vi "JSON2 speed.vi"() -> ()   [LabVIEW 2017] (continued)
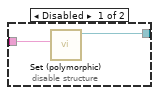
[diagram p2: hidden frame]
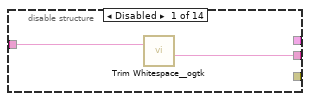
[diagram p3: hidden frame]
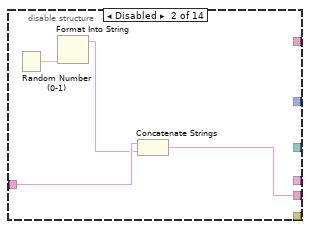
[diagram p4: hidden frame]
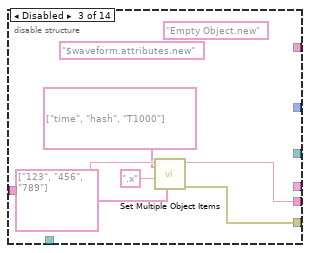
[diagram p5: hidden frame]
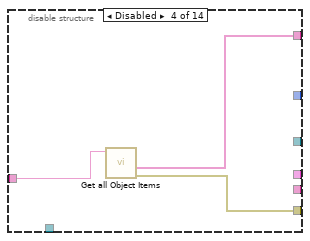
[diagram p6: hidden frame]
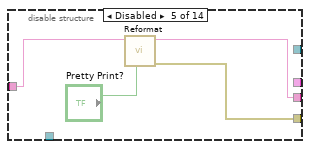
[diagram p7: hidden frame]
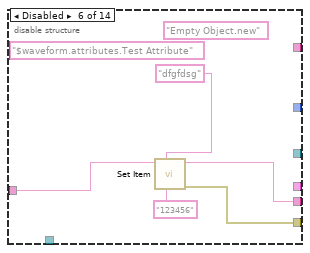
[diagram p8: hidden frame]
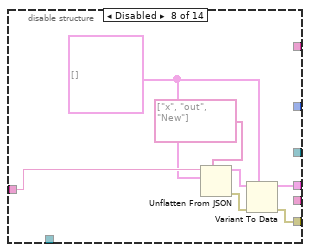
[diagram p9: hidden frame]
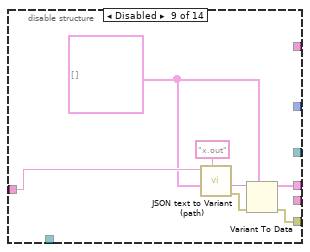
[diagram p10: hidden frame]
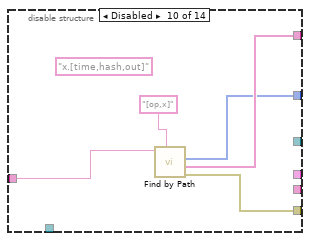
[diagram p11: hidden frame]
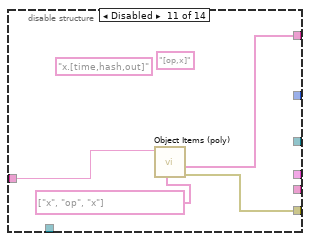
[diagram p12: hidden frame]
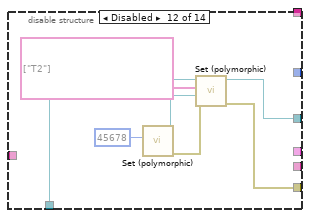
[diagram p13: hidden frame]
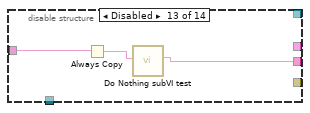
[diagram p14: hidden frame]
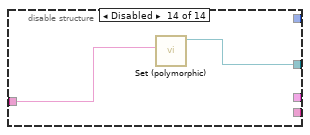
[diagram p15: hidden frame]
\\n[caliper] [performing additional measurement with scale 1.00]\\n[caliper] [running trial with 1623823839 reps]\\n[caliper] [starting measured section]\\n[caliper] [done measured section]\\n[caliper] [took 0.61 nanoseconds per rep]\\n\"}}},{\"k\":{\"variables\":{\"vm\":\"java\",\"trial\":\"0\",\"benchmark\":\"ToArray\",\"size\":\"300\"}},\"v\":{\"measurementSetMap\":{\"TIME\":{\"measurements\":[{\"raw\":239.58869988386775,\"processed\":239.58869988386775,\"unitNames\":{\"ns\":1,\"s\":1000000000,\"ms\":1000000,\"us\":1000}},{\"raw\":235.73190589527383,\"processed\":235.73190589527383,\"unitNames\":{\"ns\":1,\"s\":1000000000,\"ms\":1000000,\"us\":1000}},{\"raw\":237.79040875271875,\"processed\":237.79040875271875,\"unitNames\":{\"ns\":1,\"s\":1000000000,\"ms\":1000000,\"us\":1000}}],\"unitNames\":{\"ns\":1,\"s\":1000000000,\"ms\":1000000,\"us\":1000},\"systemOutCharCount\":0,\"systemErrCharCount\":0}},\"eventLogMap\":{\"TIME\":\"starting Scenario{vm\\u003djava, trial\\u003d0, benchmark\\u003dToArray, size\\u003d300}\\n[caliper] [starting warmup]\\n[caliper] [starting measured section]\\n[caliper] [done measured section]\\n[caliper] [starting measured section]\\n[caliper] [done measured section]\\n[caliper] [starting measured section]\\n[caliper] [done measured section]\\n[caliper] [starting measured section]\\n[caliper] [done measured section]\\n[caliper] [starting measured section]\\n[caliper] [done measured section]\\n[caliper] [starting measured section]\\n[caliper] [done measured section]\\n[caliper] [starting measured section]\\n[caliper] [done measured section]\\n[caliper] [starting measured section]\\n[caliper] [done measured section]\\n[caliper] [starting measured section]\\n[caliper] [done measured section]\\n[caliper] [starting measured section]\\n[caliper] [done measured section]\\n[caliper] [starting measured section]\\n[caliper] [done measured section]\\n[caliper] [starting measured section]\\n[caliper] [done measured section]\\n[caliper] [starting measured section]\\n[caliper] [done measured section]\\n[caliper] [starting measured section]\\n[caliper] [done measured section]\\n[caliper] [starting measured section]\\n[caliper] [done measured section]\\n[caliper] [starting measured section]\\n[caliper] [done measured section]\\n[caliper] [starting measured section]\\n[caliper] [done measured section]\\n[caliper] [starting measured section]\\n[caliper] [done measured section]\\n[caliper] [starting measured section]\\n[caliper] [done measured section]\\n[caliper] [starting measured section]\\n[caliper] [done measured section]\\n[caliper] [starting measured section]\\n[caliper] [done measured section]\\n[caliper] [starting measured section]\\n[caliper] [done measured section]\\n[caliper] [starting measured section]\\n[caliper] [done measured section]\\n[caliper] [starting measured section]\\n[caliper] [done measured section]\\n[caliper] [ending warmup]\\n[caliper] [measuring nanos per rep with scale 1.00]\\n[caliper] [running trial with 4069498 reps]\\n[caliper] [starting measured section]\\n[caliper] [done measured section]\\n[caliper] [took 239.59 nanoseconds per rep]\\n[caliper] [measuring nanos per rep with scale 0.50]\\n[caliper] [running trial with 2086909 reps]\\n[caliper] [starting measured section]\\n[caliper] [done measured section]\\n[caliper] [took 235.73 nanoseconds per rep]\\n[caliper] [measuring nanos per rep with scale 1.50]\\n[caliper] [running trial with 6260729 reps]\\n[caliper] [starting measured section]\\n[caliper] [done measured section]\\n[caliper] [took 237.79 nanoseconds per rep]\\n\"}}},{\"k\":{\"variables\":{\"vm\":\"java\",\"trial\":\"0\",\"benchmark\":\"ToArrayWithNewArray\",\"size\":\"300\"}},\"v\":{\"measurementSetMap\":{\"TIME\":{\"measurements\":[{\"raw\":529.4722583654205,\"processed\":529.4722583654205,\"unitNames\":{\"ns\":1,\"s\":1000000000,\"ms\":1000000,\"us\":1000}},{\"raw\":582.2171589349554,\"processed\":582.2171589349554,\"unitNames\":{\"ns\":1,\"s\":1000000000,\"ms\":1000000,\"us\":1000}},{\"raw\":518.510819767957,\"processed\":518.510819767957,\"unitNames\":{\"ns\":1,\"s\":1000000000,\"ms\":1000000,\"us\":1000}},{\"raw\":525.7898498045982,\"processed\":525.7898498045982,\"unitNames\":{\"ns\":1,\"s\":1000000000,\"ms\":1000000,\"us\":1000}},{\"raw\":520.3325181225125,\"processed\":520.3325181225125,\"unitNames\":{\"ns\":1,\"s\":1000000000,\"ms\":1000000,\"us\":1000}},{\"raw\":518.0572592502779,\"processed\":518.0572592502779,\"unitNames\":{\"ns\":1,\"s\":1000000000,\"ms\":1000000,\"us\":1000}},{\"raw\":518.892043778886,\"processed\":518.892043778886,\"unitNames\":{\"ns\":1,\"s\":1000000000,\"ms\":1000000,\"us\":1000}},{\"raw\":519.929733733685,\"processed\":519.929733733685,\"unitNames\":{\"ns\":1,\"s\":1000000000,\"ms\":1000000,\"us\":1000}},{\"raw\":517.0482058037575,\"processed\":517.0482058037575,\"unitNames\":{\"ns\":1,\"s\":1000000000,\"ms\":1000000,\"us\":1000}},{\"raw\":523.5689942091617,\"processed\":523.5689942091617,\"unitNames\":{\"ns\":1,\"s\":1000000000,\"ms\":1000000,\"us\":1000}}],\"unitNames\":{\"ns\":1,\"s\":1000000000,\"ms\":1000000,\"us\":1000},\"systemOutCharCount\":0,\"systemErrCharCount\":0}},\"eventLogMap\":{\"TIME\":\"starting Scenario{vm\\u003djava, trial\\u003d0, benchmark\\u003dToArrayWithNewArray, size\\u003d300}\\n[caliper] [starting warmup]\\n[caliper] [starting measured section]\\n[caliper] [done measured section]\\n[caliper] [starting measured section]\\n[caliper] [done measured section]\\n[caliper] [starting measured section]\\n[caliper] [done measured section]\\n[caliper] [starting measured section]\\n[caliper] [done measured section]\\n[caliper] [starting measured section]\\n[caliper] [done measured section]\\n[caliper] [starting measured section]\\n[caliper] [done measured section]\\n[caliper] [starting measured section]\\n[caliper] [done measured section]\\n[caliper] [starting measured section]\\n[caliper] [done measured section]\\n[caliper] [starting measured section]\\n[caliper] [done measured section]\\n[caliper] [starting measured section]\\n[caliper] [done measured section]\\n[caliper] [starting measured section]\\n[caliper] [done measured section]\\n[caliper] [starting measured section]\\n[caliper] [done measured section]\\n[caliper] [starting measured section]\\n[caliper] [done measured section]\\n[caliper] [starting measured section]\\n[caliper] [done measured section]\\n[caliper] [starting measured section]\\n[caliper] [done measured section]\\n[caliper] [starting measured section]\\n[caliper] [done measured section]\\n[caliper] [starting measured section]\\n[caliper] [done measured section]\\n[caliper] [starting measured section]\\n[caliper] [done measured section]\\n[caliper] [starting measured section]\\n[caliper] [done measured section]\\n[caliper] [starting measured section]\\n[caliper] [done measured section]\\n[caliper] [starting measured section]\\n[caliper] [done measured section]\\n[caliper] [starting measured section]\\n[caliper] [done measured section]\\n[caliper] [starting measured section]\\n[caliper] [done measured section]\\n[caliper] [ending warmup]\\n[caliper] [measuring nanos per rep with scale 1.00]\\n[caliper] [running trial with 1886785 reps]\\n[caliper] [starting measured section]\\n[caliper] [done measured section]\\n[caliper] [took 529.47 nanoseconds per rep]\\n[caliper] [measuring nanos per rep with scale 0.50]\\n[caliper] [running trial with 944336 reps]\\n[caliper] [starting measured section]\\n[caliper] [done measured section]\\n[caliper] [took 582.22 nanoseconds per rep]\\n[caliper] [measuring nanos per rep with scale 1.50]\\n[caliper] [running trial with 2833009 reps]\\n[caliper] [starting measured section]\\n[caliper] [done measured section]\\n[caliper] [took 518.51 nanoseconds per rep]\\n[caliper] [performing additional measurement with scale 1.00]\\n[caliper] [running trial with 1888673 reps]\\n[caliper] [starting measured section]\\n[caliper] [done measured section]\\n[caliper] [took 525.79 nanoseconds per rep]\\n[caliper] [performing additional measurement with scale 1.00]\\n[caliper] [running trial with 1888673 reps]\\n[caliper] [starting measured section]\\n[caliper] [done measured section]\\n[caliper] [took 520.33 nanoseconds per rep]\\n[caliper] [performing additional measurement with scale 1.00]\\n[caliper] [running trial with 1888673 reps]\\n[caliper] [starting measured section]\\n[caliper] [done measured section]\\n[caliper] [took 518.06 nanoseconds per rep]\\n[caliper] [performing additional measurement with scale 1.00]\\n[caliper] [running trial with 1888673 reps]\\n[caliper] [starting measured section]\\n[caliper] [done measured section]\\n[caliper] [took 518.89 nanoseconds per rep]\\n[caliper] [performing additional measurement with scale 1.00]\\n[caliper] [running trial with 1888673 reps]\\n[caliper] [starting measured section]\\n[caliper] [done measured section]\\n[caliper] [took 519.93 nanoseconds per rep]\\n[caliper] [performing additional measurement with scale 1.00]\\n[caliper] [running trial with 1888673 reps]\\n[caliper] [starting measured section]\\n[caliper] [done measured section]\\n[caliper] [took 517.05 nanoseconds per rep]\\n[caliper] [performing additional measurement with scale 1.00]\\n[caliper] [running trial with 1888673 reps]\\n[caliper] [starting measured section]\\n[caliper] [done measured section]\\n[caliper] [took 523.57 nanoseconds per rep]\\n\"}}},{\"k\":{\"variables\":{\"vm\":\"java\",\"trial\":\"0\",\"benchmark\":\"ToArrayWithNewEmptyArray\",\"size\":\"300\"}},\"v\":{\"measurementSetMap\":{\"TIME\":{\"measurements\":[{\"raw\":375.6254268489594,\"processed\":375.6254268489594,\"unitNames\":{\"ns\":1,\"s\":1000000000,\"ms\":1000000,\"us\":1000}},{\"raw\":383.4748815464953,\"processed\":383.4748815464953,\"unitNames\":{\"ns\":1,\"s\":1000000000,\"ms\":1000000,\"us\":1000}},{\"raw\":379.36944722198643,\"processed\":379.36944722198643,\"unitNames\":{\"ns\":1,\"s\":1000000000,\"ms\":1000000,\"us\":1000}},{\"raw\":370.71310099142596,\"processed\":370.71310099142596,\"unitNames\":{\"ns\":1,\"s\":1000000000,\"ms\":1000000,\"us\":1000}},{\"raw\":376.60096851281594,\"processed\":376.60096851281594,\"unitNames\":{\"ns\":1,\"s\":1000000000,\"ms\":1000000,\"us\":1000}},{\"raw\":392.48763365694725,\"processed\":392.48763365694725,\"unitNames\":{\"ns\":1,\"s\":1000000000,\"ms\":1000000,\"us\":1000}},{\"raw\":378.26245743223905,\"processed\":378.26245743223905,\"unitNames\":{\"ns\":1,\"s\":1000000000,\"ms\":1000000,\"us\":1000}},{\"raw\":383.08394328655794,\"processed\":383.08394328655794,\"unitNames\":{\"ns\":1,\"s\":1000000000,\"ms\":1000000,\"us\":1000}},{\"raw\":386.3181957504735,\"processed\":386.3181957504735,\"unitNames\":{\"ns\":1,\"s\":1000000000,\"ms\":1000000,\"us\":1000}},{\"raw\":376.2882306010083,\"processed\":376.2882306010083,\"unitNames\":{\"ns\":1,\"s\":1000000000,\"ms\":1000000,\"us\":1000}}],\"unitNames\":{\"ns\":1,\"s\":1000000000,\"ms\":1000000,\"us\":1000},\"systemOutCharCount\":0,\"systemErrCharCount\":0}},\"eventLogMap\":{\"TIME\":\"starting Scenario{vm\\u003djava, trial\\u003d0, benchmark\\u003dToArrayWithNewEmptyArray, size\\u003d300}\\n[caliper] [starting warmup]\\n[caliper] [starting measured section]\\n[caliper] [done measured section]\\n[caliper] [starting measured section]\\n[caliper] [done measured section]\\n[caliper] [starting measured section]\\n[caliper] [done measured section]\\n[caliper] [starting measured section]\\n[caliper] [done measured section]\\n[caliper] [starting measured section]\\n[caliper] [done measured section]\\n[caliper] [starting measured section]\\n[caliper] [done measured section]\\n[caliper] [starting measured section]\\n[caliper] [done measured section]\\n[caliper] [starting measured section]\\n[caliper] [done measured section]\\n[caliper] [starting measured section]\\n[caliper] [done measured section]\\n[caliper] [starting measured section]\\n[caliper] [done measured section]\\n[caliper] [starting measured section]\\n[caliper] [done measured section]\\n[caliper] [starting measured section]\\n[caliper] [done measured section]\\n[caliper] [starting measured section]\\n[caliper] [done measured section]\\n[caliper] [starting measured section]\\n[caliper] [done measured section]\\n[caliper] [starting measured section]\\n[caliper] [done measured section]\\n[caliper] [starting measured section]\\n[caliper] [done measured section]\\n[caliper] [starting measured section]\\n[caliper] [done measured section]\\n[caliper] [starting measured section]\\n[caliper] [done measured section]\\n[caliper] [starting measured section]\\n[caliper] [done measured section]\\n[caliper] [starting measured section]\\n[caliper] [done measured section]\\n[caliper] [starting measured section]\\n[caliper] [done measured section]\\n[caliper] [starting measured section]\\n[caliper] [done measured section]\\n[caliper] [starting measured section]\\n[caliper] [done measured section]\\n[caliper] [ending warmup]\\n[caliper] [measuring nanos per rep with scale 1.00]\\n[caliper] [running trial with 2502056 reps]\\n[caliper] [starting measured section]\\n[caliper] [done measured section]\\n[caliper] [took 375.63 nanoseconds per rep]\\n[caliper] [measuring nanos per rep with scale 0.50]\\n[caliper] [running trial with 1331113 reps]\\n[caliper] [starting measured section]\\n[caliper] [done measured section]\\n[caliper] [took 383.47 nanoseconds per rep]\\n[caliper] [measuring nanos per rep with scale 1.50]\\n[caliper] [running trial with 3993339 reps]\\n[caliper] [starting measured section]\\n[caliper] [done measured section]\\n[caliper] [took 379.37 nanoseconds per rep]\\n[caliper] [performing additional measurement with scale 1.00]\\n[caliper] [running trial with 2662226 reps]\\n[caliper] [starting measured section]\\n[caliper] [done measured section]\\n[caliper] [took 370.71 nanoseconds per rep]\\n[caliper] [performing additional measurement with scale 1.00]\\n[caliper] [running trial with 2662226 reps]\\n[caliper] [starting measured section]\\n[caliper] [done measured section]\\n[caliper] [took 376.60 nanoseconds per rep]\\n[caliper] [performing additional measurement with scale 1.00]\\n[caliper] [running trial with 2662226 reps]\\n[caliper] [starting measured section]\\n[caliper] [done measured section]\\n[caliper] [took 392.49 nanoseconds per rep]\\n[caliper] [performing additional measurement with scale 1.00]\\n[caliper] [running trial with 2662226 reps]\\n[caliper] [starting measured section]\\n[caliper] [done measured section]\\n[caliper] [took 378.26 nanoseconds per rep]\\n[caliper] [performing additional measurement with scale 1.00]\\n[caliper] [running trial with 2662226 reps]\\n[caliper] [starting measured section]\\n[caliper] [done measured section]\\n[caliper] [took 383.08 nanoseconds per rep]\\n[caliper] [performing additional measurement with scale 1.00]\\n[caliper] [running trial with 2662226 reps]\\n[caliper] [starting measured section]\\n[caliper] [done measured section]\\n[caliper] [took 386.32 nanoseconds per rep]\\n[caliper] [performing additional measurement with scale 1.00]\\n[caliper] [running trial with 2662226 reps]\\n[caliper] [starting measured section]\\n[caliper] [done measured section]\\n[caliper] [took 376.29 nanoseconds per rep]\\n\"}}},{\"k\":{\"variables\":{\"vm\":\"java\",\"trial\":\"0\",\"benchmark\":\"NewList\",\"size\":\"300\"}},\"v\":{\"measurementSetMap\":{\"TIME\":{\"measurements\":[{\"raw\":245.0469730717705,\"processed\":245.0469730717705,\"unitNames\":{\"ns\":1,\"s\":1000000000,\"ms\":1000000,\"us\":1000}},{\"raw\":240.36261220088952,\"processed\":240.36261220088952,\"unitNames\":{\"ns\":1,\"s\":1000000000,\"ms\":1000000,\"us\":1000}},{\"raw\":237.90886179758303,\"processed\":237.90886179758303,\"unitNames\":{\"ns\":1,\"s\":1000000000,\"ms\":1000000,\"us\":1000}},{\"raw\":237.64297266500853,\"processed\":237.64297266500853,\"unitNames\":{\"ns\":1,\"s\":1000000000,\"ms\":1000000,\"us\":1000}},{\"raw\":238.92836394378622,\"processed\":238.92836394378622,\"unitNames\":{\"ns\":1,\"s\":1000000000,\"ms\":1000000,\"us\":1000}},{\"raw\":240.2394376171631,\"processed\":240.2394376171631,\"unitNames\":{\"ns\":1,\"s\":1000000000,\"ms\":1000000,\"us\":1000}},{\"raw\":238.93769680336206,\"processed\":238.93769680336206,\"unitNames\":{\"ns\":1,\"s\":1000000000,\"ms\":1000000,\"us\":1000}},{\"raw\":239.9377641912837,\"processed\":239.9377641912837,\"unitNames\":{\"ns\":1,\"s\":1000000000,\"ms\":1000000,\"us\":1000}}],\"unitNames\":{\"ns\":1,\"s\":1000000000,\"ms\":1000000,\"us\":1000},\"systemOutCharCount\":0,\"systemErrCharCount\":0}},\"eventLogMap\":{\"TIME\":\"starting Scenario{vm\\u003djava, trial\\u003d0, benchmark\\u003dNewList, size\\u003d300}\\n[caliper] [starting warmup]\\n[caliper] [starting measured section]\\n[caliper] [done measured section]\\n[caliper] [starting measured section]\\n[caliper] [done measured section]\\n[caliper] [starting measured section]\\n[caliper] [done measured section]\\n[caliper] [starting measured section]\\n[caliper] [done measured section]\\n[caliper] [starting measured section]\\n[caliper] [done measured section]\\n[caliper] [starting measured section]\\n[caliper] [done measured section]\\n[caliper] [starting measured section]\\n[caliper] [done measured section]\\n[caliper] [starting measured section]\\n[caliper] [done measured section]\\n[caliper] [starting measured section]\\n[caliper] [done measured section]\\n[caliper] [starting measured section]\\n[caliper] [done measured section]\\n[caliper] [starting measured section]\\n[caliper] [done measured section]\\n[caliper] [starting measured section]\\n[caliper] [done measured section]\\n[caliper] [starting measured section]\\n[caliper] [done measured section]\\n[caliper] [starting measured section]\\n[caliper] [done measured section]\\n[caliper] [starting measured section]\\n[caliper] [done measured section]\\n[caliper] [starting measured section]\\n[caliper] [done measured section]\\n[caliper] [starting measured section]\\n[caliper] [done measured section]\\n[caliper] [starting measured section]\\n[caliper] [done measured section]\\n[caliper] [starting measured section]\\n[caliper] [done measured section]\\n[caliper] [starting measured section]\\n[caliper] [done measured section]\\n[caliper] [starting measured section]\\n[caliper] [done measured section]\\n[caliper] [starting measured section]\\n[caliper] [done measured section]\\n[caliper] [starting measured section]\\n[caliper] [done measured section]\\n[caliper] [starting measured section]\\n[caliper] [done measured section]\\n[caliper] [ending warmup]\\n[caliper] [measuring nanos per rep with scale 1.00]\\n[caliper] [running trial with 4068927 reps]\\n[caliper] [starting measured section]\\n[caliper] [done measured section]\\n[caliper] [took 245.05 nanoseconds per rep]\\n[caliper] [measuring nanos per rep with scale 0.50]\\n[caliper] [running trial with 2040425 reps]\\n[caliper] [starting measured section]\\n[caliper] [done measured section]\\n[caliper] [took 240.36 nanoseconds per rep]\\n[caliper] [measuring nanos per rep with scale 1.50]\\n[caliper] [running trial with 6121275 reps]\\n[caliper] [starting measured section]\\n[caliper] [done measured section]\\n[caliper] [took 237.91 nanoseconds per rep]\\n[caliper] [performing additional measurement with scale 1.00]\\n[caliper] [running trial with 4080850 reps]\\n[caliper] [starting measured section]\\n[caliper] [done measured section]\\n[caliper] [took 237.64 nanoseconds per rep]\\n[caliper] [performing additional measurement with scale 1.00]\\n[caliper] [running trial with 4080850 reps]\\n[caliper] [starting measured section]\\n[caliper] [done measured section]\\n[caliper] [took 238.93 nanoseconds per rep]\\n[caliper] [performing additional measurement with scale 1.00]\\n[caliper] [running trial with 4080850 reps]\\n[caliper] [starting measured section]\\n[caliper] [done measured section]\\n[caliper] [took 240.24 nanoseconds per rep]\\n[caliper] [performing additional measurement with scale 1.00]\\n[caliper] [running trial with 4080850 reps]\\n[caliper] [starting measured section]\\n[caliper] [done measured section]\\n[caliper] [took 238.94 nanoseconds per rep]\\n[caliper] [performing additional measurement with scale 1.00]\\n[caliper] [running trial with 4080850 reps]\\n[caliper] [starting measured section]\\n[caliper] [done measured section]\\n[caliper] [took 239.94 nanoseconds per rep]\\n\"}}},{\"k\":{\"variables\":{\"vm\":\"java\",\"trial\":\"0\",\"benchmark\":\"UnmodifiableWrapper\",\"size\":\"300\"}},\"v\":{\"measurementSetMap\":{\"TIME\":{\"measurements\":[{\"raw\":0.615893991252921,\"processed\":0.615893991252921,\"unitNames\":{\"ns\":1,\"s\":1000000000,\"ms\":1000000,\"us\":1000}},{\"raw\":0.6576556818031484,\"processed\":0.6576556818031484,\"unitNames\":{\"ns\":1,\"s\":1000000000,\"ms\":1000000,\"us\":1000}},{\"raw\":0.6292615009608034,\"processed\":0.6292615009608034,\"unitNames\":{\"ns\":1,\"s\":1000000000,\"ms\":1000000,\"us\":1000}},{\"raw\":0.6187731758637912,\"processed\":0.6187731758637912,\"unitNames\":{\"ns\":1,\"s\":1000000000,\"ms\":1000000,\"us\":1000}},{\"raw\":0.6277042053637764,\"processed\":0.6277042053637764,\"unitNames\":{\"ns\":1,\"s\":1000000000,\"ms\":1000000,\"us\":1000}},{\"raw\":0.6199340608988009,\"processed\":0.6199340608988009,\"unitNames\":{\"ns\":1,\"s\":1000000000,\"ms\":1000000,\"us\":1000}},{\"raw\":0.6177035558481317,\"processed\":0.6177035558481317,\"unitNames\":{\"ns\":1,\"s\":1000000000,\"ms\":1000000,\"us\":1000}},{\"raw\":0.6194245595148191,\"processed\":0.6194245595148191,\"unitNames\":{\"ns\":1,\"s\":1000000000,\"ms\":1000000,\"us\":1000}},{\"raw\":0.6237064744182478,\"processed\":0.6237064744182478,\"unitNames\":{\"ns\":1,\"s\":1000000000,\"ms\":1000000,\"us\":1000}},{\"raw\":0.6188901661592746,\"processed\":0.6188901661592746,\"unitNames\":{\"ns\":1,\"s\":1000000000,\"ms\":1000000,\"us\":1000}}],\"unitNames\":{\"ns\":1,\"s\":1000000000,\"ms\":1000000,\"us\":1000},\"systemOutCharCount\":0,\"systemErrCharCount\":0}},\"eventLogMap\":{\"TIME\":\"starting Scenario{vm\\u003djava, trial\\u003d0, benchmark\\u003dUnmodifiableWrapper, size\\u003d300}\\n[caliper] [starting warmup]\\n[caliper] [starting measured section]\\n[caliper] [done measured section]\\n[caliper] [starting measured section]\\n[caliper] [done measured section]\\n[caliper] [starting measured section]\\n[caliper] [done measured section]\\n[caliper] [starting measured section]\\n[caliper] [done measured section]\\n[caliper] [starting measured section]\\n[caliper] [done measured section]\\n[caliper] [starting measured section]\\n[caliper] [done measured section]\\n[caliper] [starting measured section]\\n[caliper] [done measured section]\\n[caliper] [starting measured section]\\n[caliper] [done measured section]\\n[caliper] [starting measured section]\\n[caliper] [done measured section]\\n[caliper] [starting measured section]\\n[caliper] [done measured section]\\n[caliper] [starting measured section]\\n[caliper] [done measured section]\\n[caliper] [starting measured section]\\n[caliper] [done measured section]\\n[caliper] [starting measured section]\\n[caliper] [done measured section]\\n[caliper] [starting measured section]\\n[caliper] [done measured section]\\n[caliper] [starting measured section]\\n[caliper] [done measured section]\\n[caliper] [starting measured section]\\n[caliper] [done measured section]\\n[caliper] [starting measured section]\\n[caliper] [done measured section]\\n[caliper] [starting measured section]\\n[caliper] [done measured section]\\n[caliper] [starting measured section]\\n[caliper] [done measured section]\\n[caliper] [starting measured section]\\n[caliper] [done measured section]\\n[caliper] [starting measured section]\\n[caliper] [done measured section]\\n[caliper] [starting measured section]\\n[caliper] [done measured section]\\n[caliper] [starting measured section]\\n[caliper] [done measured section]\\n[caliper] [starting measured section]\\n[caliper] [done measured section]\\n[caliper] [starting measured section]\\n[caliper] [done measured section]\\n[caliper] [starting measured section]\\n[caliper] [done measured section]\\n[caliper] [starting measured section]\\n[caliper] [done measured section]\\n[caliper] [starting measured section]\\n[caliper] [done measured section]\\n[caliper] [starting measured section]\\n[caliper] [done measured section]\\n[caliper] [starting measured section]\\n[caliper] [done measured section]\\n[caliper] [starting measured section]\\n[caliper] [done measured section]\\n[caliper] [starting measured section]\\n[caliper] [done measured section]\\n[caliper] [starting measured section]\\n[caliper] [done measured section]\\n[caliper] [starting measured section]\\n[caliper] [done measured section]\\n[caliper] [starting measured section]\\n[caliper] [done measured section]\\n[caliper] [ending warmup]\\n[caliper] [measuring nanos per rep with scale 1.00]\\n[caliper] [running trial with 1595861895 reps]\\n[caliper] [starting measured section]\\n[caliper] [done measured section]\\n[caliper] [took 0.62 nanoseconds per rep]\\n[caliper] [measuring nanos per rep with scale 0.50]\\n[caliper] [running trial with 811828020 reps]\\n[caliper] [starting measured section]\\n[caliper] [done measured section]\\n[caliper] [took 0.66 nanoseconds per rep]\\n[caliper] [measuring nanos per rep with scale 1.50]\\n[caliper] [running trial with 2147483647 reps]\\n[caliper] [starting measured section]\\n[caliper] [done measured section]\\n[caliper] [took 0.63 nanoseconds per rep]\\n[caliper] [performing additional measurement with scale 1.00]\\n[caliper] [running trial with 1623656041 reps]\\n[caliper] [starting measured section]\\n[caliper] [done measured section]\\n[caliper] [took 0.62 nanoseconds per rep]\\n[caliper] [performing additional measurement with scale 1.00]\\n[caliper] [running trial with 1623656041 reps]\\n[caliper] [starting measured section]\\n[caliper] [done measured section]\\n[caliper] [took 0.63 nanoseconds per rep]\\n[caliper] [performing additional measurement with scale 1.00]\\n[caliper] [running trial with 1623656041 reps]\\n[caliper] [starting measured section]\\n[caliper] [done measured section]\\n[caliper] [took 0.62 nanoseconds per rep]\\n[caliper] [performing additional measurement with scale 1.00]\\n[caliper] [running trial with 1623656041 reps]\\n[caliper] [starting measured section]\\n[caliper] [done measured section]\\n[caliper] [took 0.62 nanoseconds per rep]\\n[caliper] [performing additional measurement with scale 1.00]\\n[caliper] [running trial with 1623656041 reps]\\n[caliper] [starting measured section]\\n[caliper] [done measured section]\\n[caliper] [took 0.62 nanoseconds per rep]\\n[caliper] [performing additional measurement with scale 1.00]\\n[caliper] [running trial with 1623656041 reps]\\n[caliper] [starting measured section]\\n[caliper] [done measured section]\\n[caliper] [took 0.62 nanoseconds per rep]\\n[caliper] [performing additional measurement with scale 1.00]\\n[caliper] [running trial with 1623656041 reps]\\n[caliper] [starting measured section]\\n[caliper] [done measured section]\\n[caliper] [took 0.62 nanoseconds per rep]\\n\"}}}]},\"environment\":{\"propertyMap\":{\"jre.vmname\":\"Java HotSpot(TM) 64-Bit Server VM\",\"host.cpu.names\":\"[Intel(R) Core(TM) i5-3320M CPU @ 2.60GHz x 4]\",\"jre.version\":\"1.6.0_32-ea-b03\",\"host.cpu.cores\":\"[2 x 4]\",\"jre.availableProcessors\":\"4\",\"os.name\":\"Linux\",\"jre.vmversion\":\"20.7-b02\",\"host.memory.swap\":\"[6183932 kB]\",\"os.version\":\"3.5.0-25-generic\",\"host.cpu.cachesize\":\"[3072 KB x 4]\",\"host.cpus\":\"4\",\"host.name\":\"kelvin\",\"os.arch\":\"amd64\",\"host.memory.physical\":\"[7871592 kB]\"}}}"
  n1 = String Length(string=w1) -> (length=→"length":i32)
  n2 = disable-structure shown="Enabled" {
    disable-tunnel: [w13 _] -> w2
    disable-tunnel: w1 -> [w12 _]
    frame Disabled {
      n3 = call-poly <vilib>:"Set (polymorphic).vi"("JSON stream"=w12) -> ("JSON Value out"=w13:refnum<class "JSON Value.lvclass">)  [unwired: 8 in, 2 out]
    }
    frame Enabled {
    }
  }
  n4 = for {
    N: 10 -> [_]
    tunnel: [w25] -> w9 mode=indexing
    tunnel: w1 -> [w19]
    tunnel: [w24] -> w4 mode=indexing
    tunnel: w2 -> [w18]
    i -> [w17]
    (unwired) string[] ["waveform", "attributes", "New"] ("Name Array")
    (unwired) "waveform.attributes.Test Attribute" ("Item Path")
    (unwired) "$waveform.attributes.Test Attribute" ("Item Path")
    (unwired) "{\"2\":2%s}  D" ("format string")
    (unwired) ",\"a\":1"
    n5 = Initialize Array(" ", 1000000 ("dimension size")) -> (w27:string[])
    n6 = Concatenate Strings(w27) -> (w26:string)
    n7 = Format Into String(format string="%s123", w26) -> ()  [unwired: 2 in, 2 out]
    n8 = Always Copy(1:w19) -> (0:w20:string)
    n9 = flat-sequence {
      tunnel: [w34] -> w23
      tunnel: w20 -> [_]
      frame #0 {
        n10 = Wait (ms)(milliseconds to wait=u32 0) -> (millisecond timer value=w34:u32)
      }
    }
    n11 = flat-sequence {
      tunnel: [w46] -> w32
      tunnel: [w45] -> w31
      tunnel: w20 -> [w44]
      tunnel: [w43] -> _
      tunnel: w23 -> [w42]
      tunnel: [w41] -> w22
      tunnel: [w40] -> w21
      tunnel: w18 -> [w39]
      tunnel: [w38] -> w16
      tunnel: [w37] -> w14
      tunnel: [w36] -> w15
      frame #0 {
        n12 = flat-sequence {
          tunnel: [w114] -> w43
          tunnel: w44 -> [w114]
          tunnel: [w113] -> w45
          tunnel: w42 -> [_]
          frame #0 {
            n13 = call <vilib>:"High Resolution Relative Seconds.vi"() -> ("relative seconds"=w113:dbl)
          }
        }
        n14 = disable-structure shown="Enabled" {
          disable-tunnel: w43 -> [w49 w53 w59 w62 w66 w71 w75 w82 w89 w94 w98 _ w106 w110]
          disable-tunnel: [w48 w52 w58 _ w64 w70 w72 _ _ _ _ _ w108 _] -> w47
          disable-tunnel: [_ _ _ _ _ _ _ _ _ _ _ w101 _ w109] -> _
          disable-tunnel: [_ _ w56 w61 w65 w68 w74 w77 w83 w93 w97 w99 _ _] -> w41
          disable-tunnel: w39 -> [_ _ _ _ _ _ _ _ _ _ _ w104 _ _]
          disable-tunnel: [_ _ _ w60 _ _ _ _ _ w91 w96 _ _ _] -> w38
          disable-tunnel: [_ _ _ _ _ _ _ _ _ w90 _ _ _ _] -> w37
          disable-tunnel: [_ _ _ _ _ _ _ w80 w87 _ _ _ _ _] -> w36
          frame Disabled {
            n15 = call-poly <userlib>:"Trim Whitespace__ogtk.vi"("String in"=w49) -> ("String out"=w48:string)  [unwired: 6 in]
          }
          frame Disabled {
            n16 = Random Number (0-1)() -> (number: 0 to 1=w51:dbl)
            n17 = Format Into String(w51) -> (resulting string=w50:string)  [unwired: 3 in, 1 out]
            n18 = Concatenate Strings(w53, w50) -> (w52:string)
          }
          frame Disabled {
            (unwired) "Empty Object.new" ("Item Path")
            (unwired) "$waveform.attributes.new" ("Item Path")
            n19 = call "Set Multiple Object Items.vi"("Item Names"=string[] ["123", "456", "789"] ("Name Array"), "$Path or Item Name"=string[] ["time", "hash", "T1000"] ("Name Array"), "JSON Items"=".x" ("JSON to Insert"), "JSON"=w59) -> ("error out"=w56:errorcluster, "<JSON>"=w58:string)  [unwired: 5 in]
          }
          frame Disabled {
            n20 = call "Get all Object Items.vi"("JSON"=w62) -> ("error out"=w61:errorcluster, "<JSON>"=w60:string[])  [unwired: 7 in, 2 out]
          }
          frame Disabled {
            n21 = call "Reformat.vi"("Pretty Print Levels"="Pretty Print?", "Input String"=w66) -> ("error out"=w65:errorcluster, "<JSON>First JSON Value"=w64:string)  [unwired: 5 in, 2 out]
          }
          frame Disabled {
            (unwired) "Empty Object.new" ("Item Path")
            (unwired) "$waveform.attributes.Test Attribute" ("Item Path")
            n22 = call "Set Item.vi"(5:"123456" ("JSON to Insert"), "$Path or Item Name"="dfgfdsg" ("Item Path"), "JSON"=w71) -> ("error out"=w68:errorcluster, "<JSON>"=w70:string)  [unwired: 5 in, 1 out]
          }
          frame Enabled {
            (unwired) "x.[time,hash,out]" ("Item Path")
            n23 = call-poly "Find by Path.vi"("$Path or Item Name"="dfgdf" ("Item Path"), "JSON"=w75) -> ("error out"=w74:errorcluster, "<JSON>Item"=w72:string)  [unwired: 6 in, 2 out]
          }
          frame Disabled {
            w79 = cluster{"spent":bool, "value":i32}[] []
            n24 = Unflatten From JSON(path=string[] ["x", "out", "New"] ("Name Array"), JSON string=w82, type and defaults=w79) -> (value=w81:cluster{"spent":bool, "value":i32}[], error out=w78:errorcluster)  [unwired: 4 in]
            n25 = Variant To Data(error in=w78, type=w79, Variant=w81) -> (data=w80:cluster{"spent":bool, "value":i32}[], error out=w77:errorcluster)
          }
          frame Disabled {
            w86 = cluster{"spent":bool, "value":i32}[] []
            n26 = call "JSON text to Variant (path).vi"("Item Path"="x.out", "Variant (Data Type)"=w86, "JSON"=w89) -> ("error out"=w84:errorcluster, "Variant out"=w88:variant)  [unwired: 6 in, 1 out]
            n27 = Variant To Data(error in=w84, type=w86, Variant=w88) -> (data=w87:cluster{"spent":bool, "value":i32}[], error out=w83:errorcluster)
          }
          frame Disabled {
            (unwired) "x.[time,hash,out]" ("Item Path")
            n28 = call-poly "Find by Path.vi"("$Path or Item Name"="[op,x]" ("Item Path"), "JSON"=w94) -> ("error out"=w93:errorcluster, "<JSON>Items"=w91:string[], "Offsets"=w90:i32[])  [unwired: 6 in, 1 out]
          }
          frame Disabled {
            (unwired) "x.[time,hash,out]" ("Item Path")
            (unwired) "[op,x]" ("Item Path")
            n29 = call-poly "Object Items (poly).vi"("Item Names"=string[] ["x", "op", "x"], "JSON"=w98) -> ("error out"=w97:errorcluster, "<JSON>"=w96:string[])  [unwired: 7 in, 1 out]
          }
          frame Disabled {
            n30 = call-poly <vilib>:"Set (polymorphic).vi"("Numeric"=i64 45678) -> ("error out"=w100:errorcluster, "JSON Scalar out"=w103:refnum<class "JSON Scalar.lvclass">)  [unwired: 9 in]
            n31 = call-poly <vilib>:"Set (polymorphic).vi"("error in (no error)"=w100, "Value"=w103, "Name Array"=string[] ["T2"], "JSON Value In"=w104) -> ("error out"=w99:errorcluster, "JSON Value Out"=w101:refnum<class "JSON Value.lvclass">)  [unwired: 5 in, 1 out]
          }
          frame Disabled {
            n32 = Always Copy(1:w106) -> (0:w107:string)
            n33 = call "Do Nothing subVI test.vi"("String"=w107) -> ("String 2"=w108:string)  [unwired: 10 in]
          }
          frame Disabled {
            n34 = call-poly <vilib>:"Set (polymorphic).vi"("JSON stream"=w110) -> ("JSON Value out"=w109:refnum<class "JSON Value.lvclass">)  [unwired: 8 in, 2 out]
          }
        }
        n35 = flat-sequence {
          tunnel: [w112] -> w40
          tunnel: w47 -> [w112]
          tunnel: [w111] -> w46
          frame #0 {
            n36 = call <vilib>:"High Resolution Relative Seconds.vi"() -> ("relative seconds"=w111:dbl)
          }
        }
      }
    }
    n37 = String Length(string=w19) -> (length=w29:i32)
    n38 = Subtract(x=w32, y=w31) -> (x-y=w24:dbl)
    n39 = Divide(x=w24, y=w29) -> (x/y=w25:dbl)
    "String out" <- w21
    "error out" <- w22
    "Numeric" <- w17
    "<JSON>" <- w16
    "Variant out" <- w15
    "Offsets" <- w14
  }
  "per char" <- w9
  "time" <- w4
  n40 = Array Subset(array=w9, index=1) -> (w7:dbl[])  [unwired: 1 in]
  n41 = call <vilib>:"Measures of Mean.vi"("type"=w3, "x array"=w7) -> ("mean value"=→"mean":dbl)  [unwired: 8 in, 1 out]
  n42 = call <vilib>:"Measures of Mean.vi"("type"=w3, "x array"=w4) -> ("mean value"=→"mean 2":dbl)  [unwired: 8 in, 1 out]
